vi "Camera Messenger.vi"(0 "Notifier Name":string, 2 "General Camera Actions":T3, 5 "Exposure Time (s)":dbl, 7 "Save Path":path, 9 "No. of Frames":u32, 11 "Camera ROI":T1, 12 "Cooler On/Off":bool, 13 "Defect Correction On/Off":bool, 14 "Fan On/Off":bool) -> (3 "Current Exposure Time (s)":dbl, 4 "Notifier Name Dup":string, 6 "Running?":bool, 8 "Camera ROI":T1, 10 "Current Frame":u32, 15 "Image Ref":T2)   [LabVIEW 2016]
uses:
  Camera Controls/Generic Camera Actions.ctl
  Camera Controls/Generic Camera ROI.ctl
  <vilib>/vision/Image Controls.llb/IMAQ Image.ctl
  Hardware Configuration/Hardware Configuration Controls/Company.ctl
  Hamamatsu/Orca Flash/Orca Flash Controls/Orca Flash ROI.ctl
  Hamamatsu/Orca Flash/Orca Flash Controls/Orca Flash Parameters.ctl
  Hamamatsu/Orca Flash/Orca Flash Controls/Orca Flash Parameter List.ctl
  Hamamatsu/Orca Flash/Orca Flash Controls/Orca Flash Actions.ctl
  IDS/IDS Controls/IDS ROI.ctl
  IDS/IDS Controls/IDS Parameters.ctl
  IDS/IDS Controls/IDS Parameter List.ctl
  IDS/IDS Controls/IDS Actions.ctl
  Photometrics/Prime BSI/Prime BSI Controls/Prime ROI.ctl
  Photometrics/Prime BSI/Prime BSI Controls/Prime Parameters.ctl
  Photometrics/Prime BSI/Prime BSI Controls/Prime Parameter List.ctl
  Photometrics/Prime BSI/Prime BSI Controls/Prime Actions.ctl
  Camera Controls/Camera IMAQ Key Info.ctl
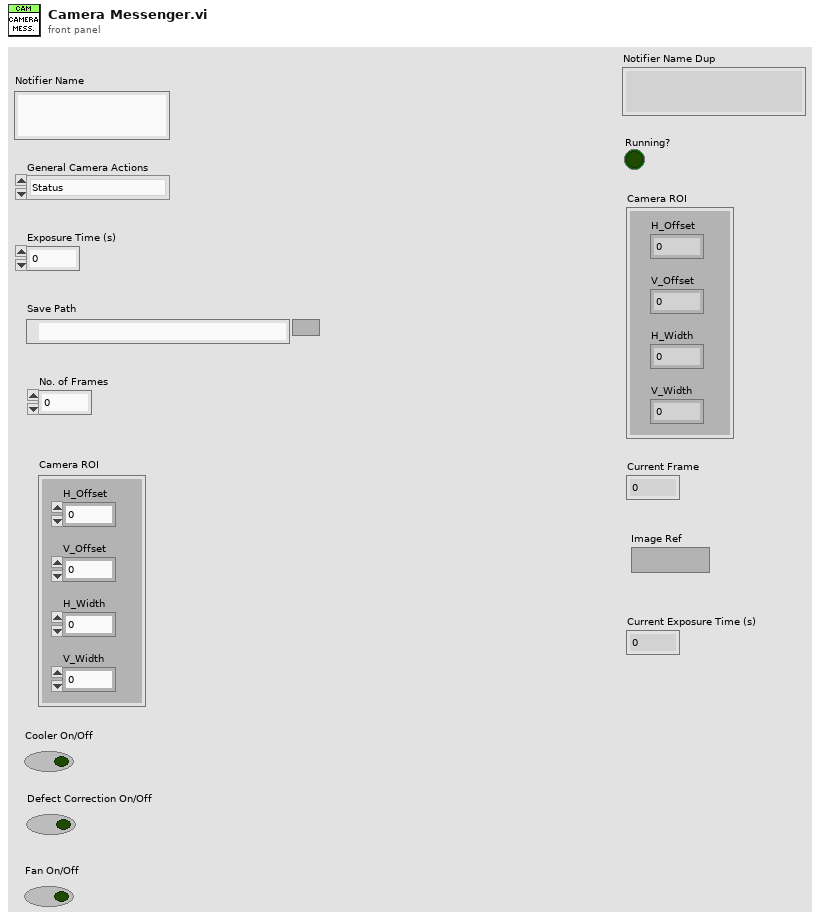
[diagram p1: front panel]
types:
  T1 = typedef "Generic Camera ROI.ctl" = cluster{"H_Offset":u16, "V_Offset":u16, "H_Width":u16, "V_Width":u16}
  T2 = typedef "IMAQ Image.ctl" = refnum<image>
  T3 = typedef "Generic Camera Actions.ctl" = enum16{"Status", "Ext trigger\n", "Live Preview", "Capture", "Abort", "Set Exposure Time (s)", "Get Exposure Time (s)", "Record Settings", "Set ROI", "Get ROI", "Defect Correction On/Off", "Cooler On/Off", "Fan On/Off", "Quti"}
  T4 = typedef "Company.ctl" = enum16{"AA Opto Electronic", "ASI", "Coherent", "CVI", "DAQmx", "Hamamatsu", "IDS", "Mad City Labs", "Marzhauser", "Measurement Computing", "MPB Com", "Photometrics", "PI", "Prior", "Thorlabs"}
  T5 = typedef "Orca Flash Parameters.ctl" = cluster{"Value":dbl, "Parameter":T6}
  T6 = typedef "Orca Flash Parameter List.ctl" = u32
  T7 = typedef "Orca Flash ROI.ctl" = cluster{"H Offset":i32, "V Offset":i32, "H Width":i32, "V Width":i32}
  T8 = typedef "Orca Flash Actions.ctl" = enum16{"IDLE", "PREVIEW", "RECORD", "Record Settings", "SETPARAM", "GETPARAM", "SETROI", "GETROI", "PROGRESSIVE MODE", "AREA MODE", "STATUS", "Trigger synchronous", "Trigger internal", "QUIT"}
  T9 = typedef "IDS Parameter List.ctl" = enum16{"Exposure Time (s)"}
  T10 = typedef "IDS Parameters.ctl" = cluster{"Parameter":T9, "Value":dbl}
  T11 = typedef "IDS ROI.ctl" = cluster{"H Offset":i32, "V Offset":i32, "H Width":i32, "V Width":i32}
  T12 = typedef "IDS Actions.ctl" = enum16{"Error Check", "Initialize", "Preview", "Record", "Abort", "Record Settings", "Set Parameter", "Get Parameter", "Set ROI", "Get ROI", "Status", "Quit"}
  T13 = typedef "Prime Parameter List.ctl" = enum16{"Exposure Time (s)"}
  T14 = typedef "Prime Parameters.ctl" = cluster{"Parameter":T13, "Value":dbl}
  T15 = typedef "Prime ROI.ctl" = cluster{"X Start":u32, "X End":u32, "X Bin":u32, "Y Start":u32, "Y End":u32, "Y Bin":u32}
  T16 = typedef "Prime Actions.ctl" = enum16{"Error Check", "Initialize", "Preview", "Record", "Abort", "Record Settings", "Set Parameter", "Get Parameter", "Set ROI", "Get ROI", "Status", "Set Trigger", "Quit"}
  T17 = typedef "Camera IMAQ Key Info.ctl" = cluster{"Frame":u32, "Sensor Height":i32, "Sensor Width":i32, "ROI Height":i32, "ROI Width":i32, "ROI Enable?":bool, "Bit per Pixel":u8}
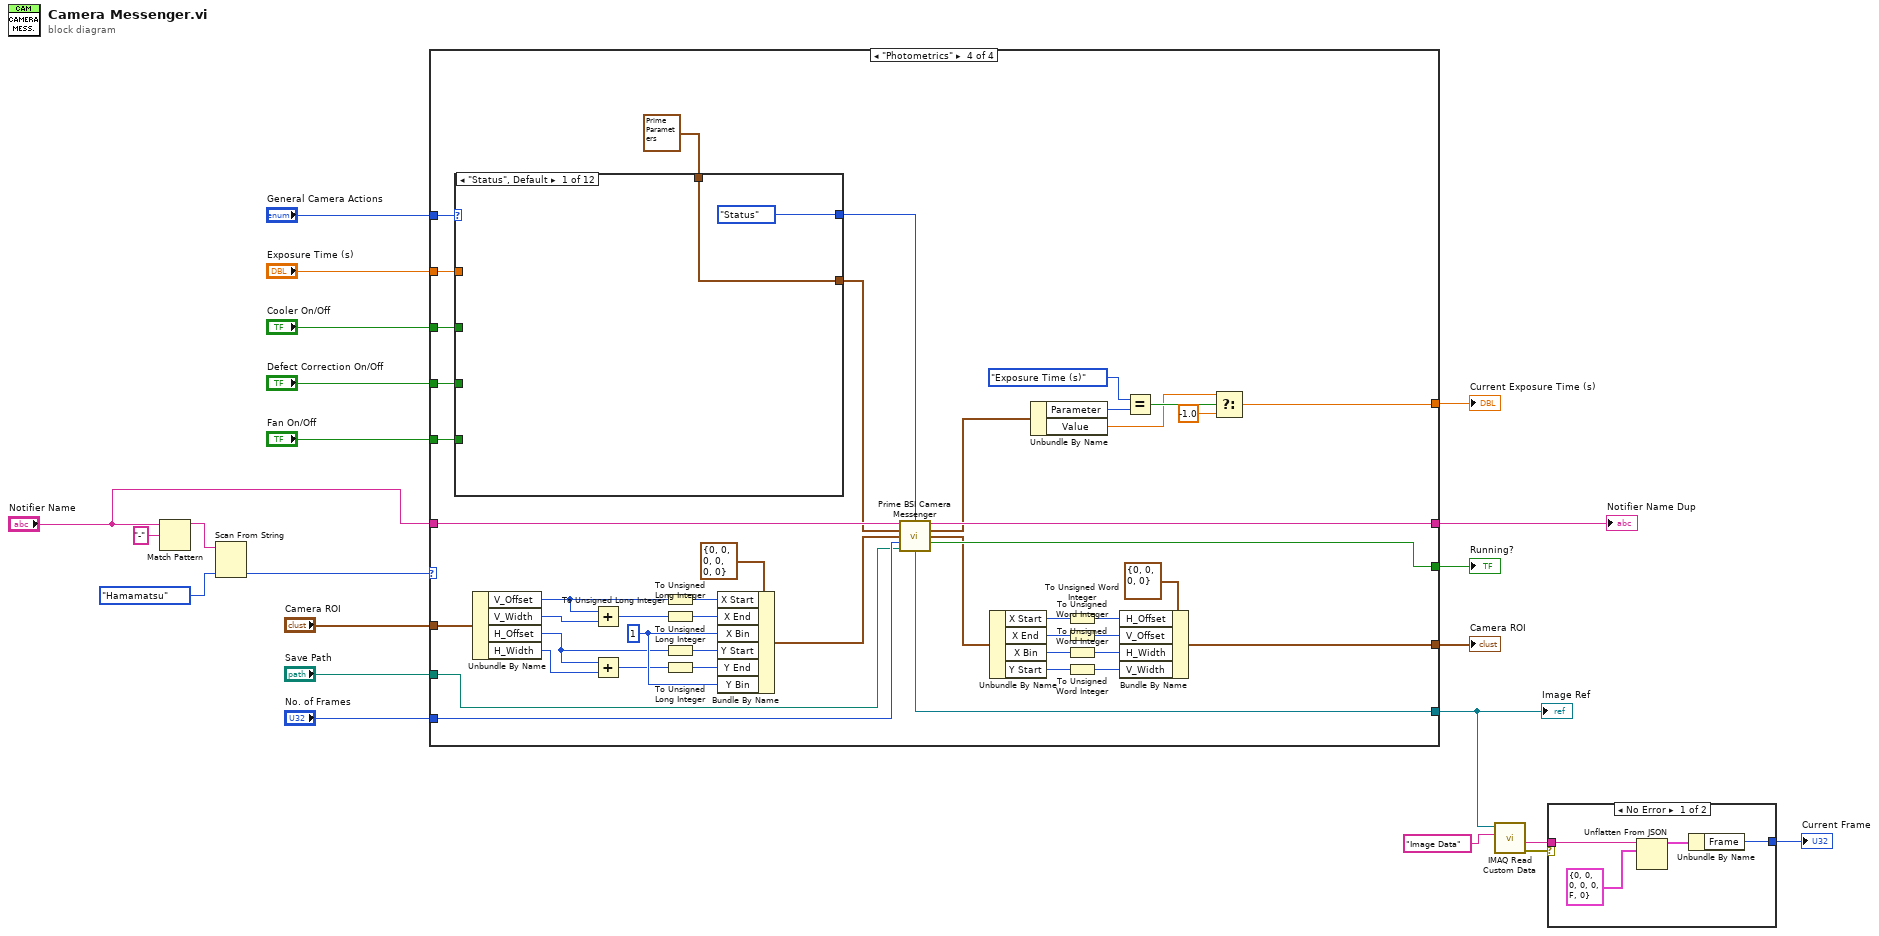
[diagram p0: block diagram]
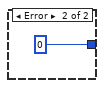
[diagram p2: hidden frame]
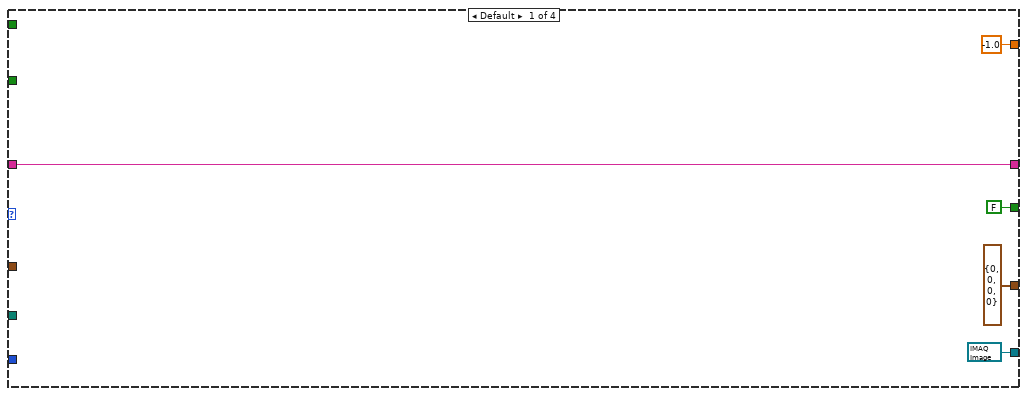
[diagram p3: hidden frame]
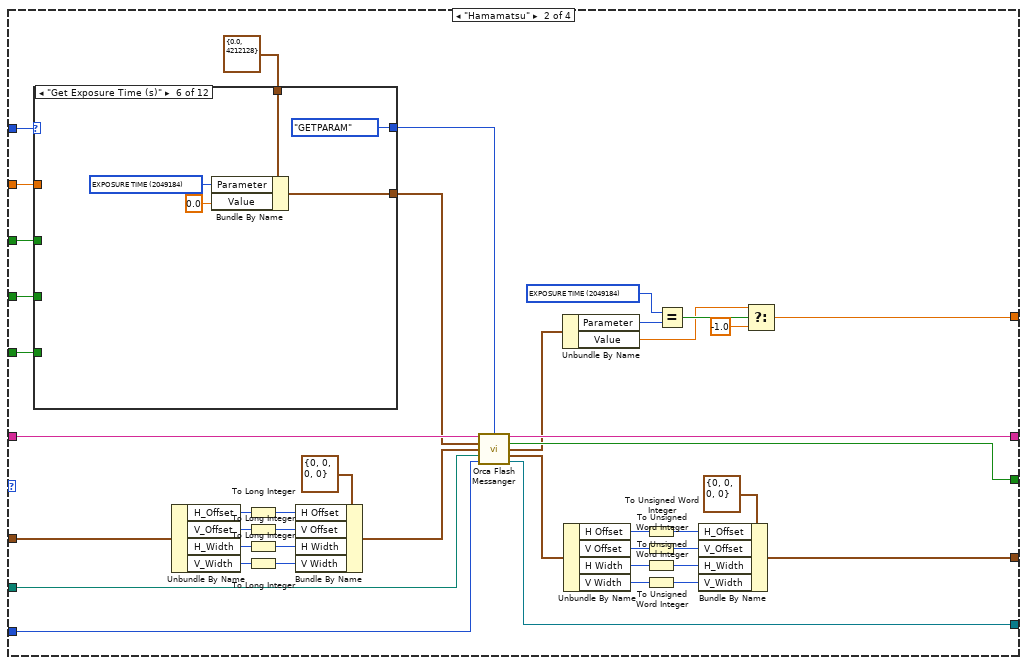
[diagram p4: hidden frame]
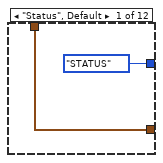
[diagram p5: hidden frame]
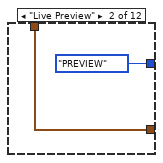
[diagram p6: hidden frame]
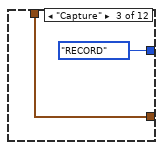
[diagram p7: hidden frame]
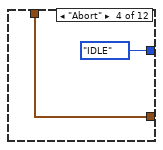
[diagram p8: hidden frame]
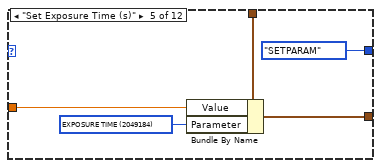
[diagram p9: hidden frame]
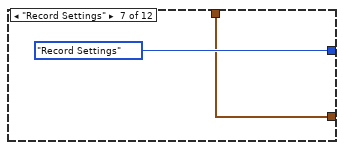
[diagram p10: hidden frame]
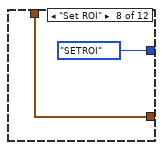
[diagram p11: hidden frame]
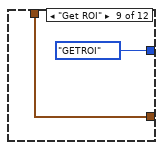
[diagram p12: hidden frame]
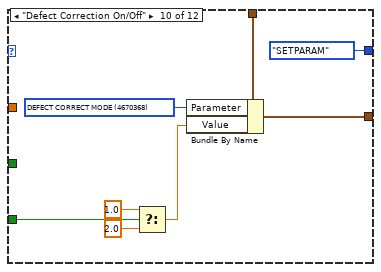
[diagram p13: hidden frame]
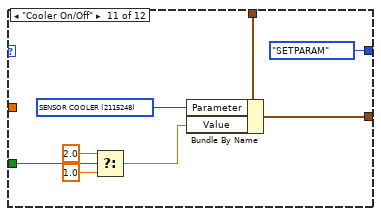
[diagram p14: hidden frame]
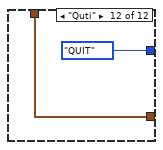
[diagram p15: hidden frame]
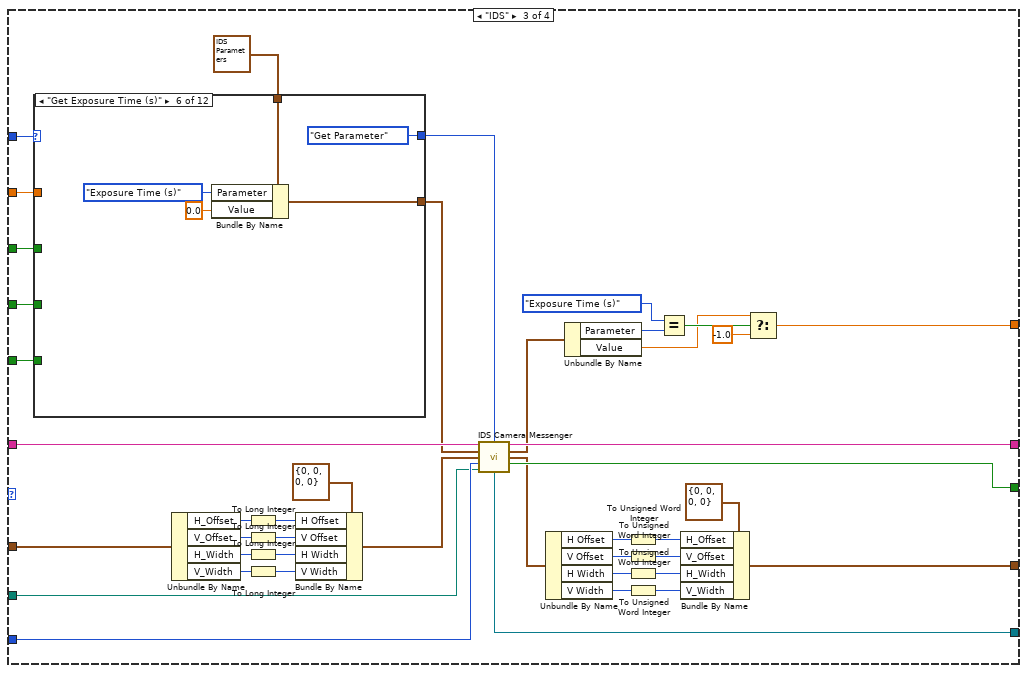
[diagram p16: hidden frame]
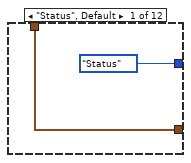
[diagram p17: hidden frame]
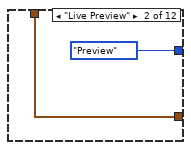
[diagram p18: hidden frame]
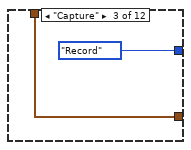
[diagram p19: hidden frame]
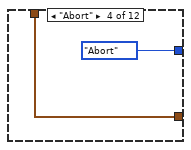
[diagram p20: hidden frame]
diagram:
  n1 = Match Pattern(string="Notifier Name", regular expression="-") -> (before substring=w19:string)  [unwired: 1 in, 3 out]
  n2 = Scan From String(input string=w19, default 1=Company."Hamamatsu" ("Company")) -> (output 1=w20:T4)  [unwired: 3 in, 3 out]
  n3 = case shown="\"Photometrics\"" w20 {
    tunnel: "Notifier Name" -> [w27 w70 w155 w231]
    tunnel: "General Camera Actions" -> [_ w55 w140 w224]
    tunnel: "No. of Frames" -> [_ w69 w154 w230]
    tunnel: "Save Path" -> [_ w68 w153 w202]
    tunnel: "Camera ROI" -> [_ w66 w151 w228]
    tunnel: [w27 w56 w141 w225] -> w14
    tunnel: "Exposure Time (s)" -> [_ w50 w136 w220]
    tunnel: "Cooler On/Off" -> [_ w54 w139 w223]
    tunnel: "Defect Correction On/Off" -> [_ w53 w138 w222]
    tunnel: "Fan On/Off" -> [_ w52 w137 w221]
    tunnel: [T2 refnum ("Image Ref") w47 w133 w217] -> w5
    tunnel: [FALSE ("Running?") w46 w132 w216] -> w9
    tunnel: [T1 {"H_Offset"=0, "V_Offset"=0, "H_Width"=0, "V_Width"=0} ("General Camera ROI") w35 w121 w205] -> w8
    tunnel: [-1.0 ("f") w29 w113 w187] -> w1
    frame Default {
    }
    frame "Hamamatsu" {
      w28 = T6 2049184 items=["SENSOR MODE"=4212128, "READOUT SPEED"=4211872, "READOUT DIRECTION"=4211904, "TRIGGER GLOBAL EXPOSURE"=2049680, "TRIGGER DELAY"=1066480, "SYNC READOUT SYSTEM BLANK"=1066528, "SENSOR COOLER"=2115248, "SENSOR COOLER STATUS"=2115280, "EXPOSURE TIME"=2049184, "DEFECT CORRECT MODE"=4670368, "BINNING"=4215968, "INTERNAL LINE SPEED"=4226000, "INTERNAL LINE INTERVAL"=4226016, "IMAGE PIXEL TYPE"=4343296, "NUMBER OF OUTPUT TRIGGER CONNECTOR"=1852320, "OUTPUT TRIGGER SOURCE[0]"=1852576, "OUTPUT TRIGGER SOURCE[1]"=1852832, "OUTPUT TRIGGER SOURCE[2]"=1853088, "OUTPUT TRIGGER POLARITY[0]"=1852592, "OUTPUT TRIGGER POLARITY[1]"=1852848, "OUTPUT TRIGGER POLARITY[2]"=1853104, "OUTPUT TRIGGER ACTIVE[0]"=1852608, "OUTPUT TRIGGER ACTIVE[1]"=1852864, "OUTPUT TRIGGER ACTIVE[2]"=1853120, "OUTPUT TRIGGER DELAY[0]"=1852624, "OUTPUT TRIGGER DELAY[1]"=1852880, "OUTPUT TRIGGER DELAY[2]"=1853136, "OUTPUT TRIGGER PERIOD[0]"=1852640, "OUTPUT TRIGGER PERIOD[1]"=1852896, "OUTPUT TRIGGER PERIOD[2]"=1853152, "OUTPUT TRIGGER KIND[0]"=1852656, "OUTPUT TRIGGER KIND[1]"=1852912, "OUTPUT TRIGGER KIND[2]"=1853168, "OUTPUT TRIGGER PRE HSYNC COUNT"=1852704] ("x")
      n4 = case shown="\"Get Exposure Time (s)\"" w55 {
        tunnel: w54 -> [_ _ _ _ _ _ _ _ _ _ w107 _]
        tunnel: w53 -> [_ _ _ _ _ _ _ _ _ w98 _ _]
        tunnel: w52 -> [_ _ _ _ _ _ _ _ _ _ _ _]
        tunnel: [Orca_Flash_Actions."STATUS" ("Camera Actions") Orca_Flash_Actions."PREVIEW" ("Camera Actions") Orca_Flash_Actions."RECORD" ("Camera Actions") Orca_Flash_Actions."IDLE" ("Camera Actions") Orca_Flash_Actions."SETPARAM" ("Camera Actions") Orca_Flash_Actions."GETPARAM" ("Camera Actions") Orca_Flash_Actions."Record Settings" ("Camera Actions") Orca_Flash_Actions."SETROI" ("Camera Actions") Orca_Flash_Actions."GETROI" ("Camera Actions") Orca_Flash_Actions."SETPARAM" ("Camera Actions") Orca_Flash_Actions."SETPARAM" ("Camera Actions") Orca_Flash_Actions."QUIT" ("Camera Actions")] -> w51
        tunnel: w50 -> [_ _ _ _ w82 _ _ _ _ _ _ _]
        tunnel: [w71 w73 w75 w77 w81 w87 w89 w91 w93 w100 w103 w112] -> w49
        tunnel: T5 {"Value"=0.0, "Parameter"=4212128} ("sCMOS Parameter") -> [w71 w73 w75 w77 w80 w88 w89 w91 w93 w101 w109 w112]
        frame "Status", Default {
        }
        frame "Live Preview" {
        }
        frame "Capture" {
        }
        frame "Abort" {
        }
        frame "Set Exposure Time (s)" {
          w79 = T6 2049184 items=["SENSOR MODE"=4212128, "READOUT SPEED"=4211872, "READOUT DIRECTION"=4211904, "TRIGGER GLOBAL EXPOSURE"=2049680, "TRIGGER DELAY"=1066480, "SYNC READOUT SYSTEM BLANK"=1066528, "SENSOR COOLER"=2115248, "SENSOR COOLER STATUS"=2115280, "EXPOSURE TIME"=2049184, "DEFECT CORRECT MODE"=4670368, "BINNING"=4215968, "INTERNAL LINE SPEED"=4226000, "INTERNAL LINE INTERVAL"=4226016, "IMAGE PIXEL TYPE"=4343296, "NUMBER OF OUTPUT TRIGGER CONNECTOR"=1852320, "OUTPUT TRIGGER SOURCE[0]"=1852576, "OUTPUT TRIGGER SOURCE[1]"=1852832, "OUTPUT TRIGGER SOURCE[2]"=1853088, "OUTPUT TRIGGER POLARITY[0]"=1852592, "OUTPUT TRIGGER POLARITY[1]"=1852848, "OUTPUT TRIGGER POLARITY[2]"=1853104, "OUTPUT TRIGGER ACTIVE[0]"=1852608, "OUTPUT TRIGGER ACTIVE[1]"=1852864, "OUTPUT TRIGGER ACTIVE[2]"=1853120, "OUTPUT TRIGGER DELAY[0]"=1852624, "OUTPUT TRIGGER DELAY[1]"=1852880, "OUTPUT TRIGGER DELAY[2]"=1853136, "OUTPUT TRIGGER PERIOD[0]"=1852640, "OUTPUT TRIGGER PERIOD[1]"=1852896, "OUTPUT TRIGGER PERIOD[2]"=1853152, "OUTPUT TRIGGER KIND[0]"=1852656, "OUTPUT TRIGGER KIND[1]"=1852912, "OUTPUT TRIGGER KIND[2]"=1853168, "OUTPUT TRIGGER PRE HSYNC COUNT"=1852704] ("Parameter")
          n5 = Bundle By Name(cluster=w80, "Value"=w82, "Parameter"=w79) -> (w81:T5)
        }
        frame "Get Exposure Time (s)" {
          w85 = T6 2049184 items=["SENSOR MODE"=4212128, "READOUT SPEED"=4211872, "READOUT DIRECTION"=4211904, "TRIGGER GLOBAL EXPOSURE"=2049680, "TRIGGER DELAY"=1066480, "SYNC READOUT SYSTEM BLANK"=1066528, "SENSOR COOLER"=2115248, "SENSOR COOLER STATUS"=2115280, "EXPOSURE TIME"=2049184, "DEFECT CORRECT MODE"=4670368, "BINNING"=4215968, "INTERNAL LINE SPEED"=4226000, "INTERNAL LINE INTERVAL"=4226016, "IMAGE PIXEL TYPE"=4343296, "NUMBER OF OUTPUT TRIGGER CONNECTOR"=1852320, "OUTPUT TRIGGER SOURCE[0]"=1852576, "OUTPUT TRIGGER SOURCE[1]"=1852832, "OUTPUT TRIGGER SOURCE[2]"=1853088, "OUTPUT TRIGGER POLARITY[0]"=1852592, "OUTPUT TRIGGER POLARITY[1]"=1852848, "OUTPUT TRIGGER POLARITY[2]"=1853104, "OUTPUT TRIGGER ACTIVE[0]"=1852608, "OUTPUT TRIGGER ACTIVE[1]"=1852864, "OUTPUT TRIGGER ACTIVE[2]"=1853120, "OUTPUT TRIGGER DELAY[0]"=1852624, "OUTPUT TRIGGER DELAY[1]"=1852880, "OUTPUT TRIGGER DELAY[2]"=1853136, "OUTPUT TRIGGER PERIOD[0]"=1852640, "OUTPUT TRIGGER PERIOD[1]"=1852896, "OUTPUT TRIGGER PERIOD[2]"=1853152, "OUTPUT TRIGGER KIND[0]"=1852656, "OUTPUT TRIGGER KIND[1]"=1852912, "OUTPUT TRIGGER KIND[2]"=1853168, "OUTPUT TRIGGER PRE HSYNC COUNT"=1852704] ("Parameter")
          n6 = Bundle By Name(cluster=w88, "Parameter"=w85, "Value"=0.0) -> (w87:T5)
        }
        frame "Record Settings" {
        }
        frame "Set ROI" {
        }
        frame "Get ROI" {
        }
        frame "Defect Correction On/Off" {
          w99 = T6 4670368 items=["SENSOR MODE"=4212128, "READOUT SPEED"=4211872, "READOUT DIRECTION"=4211904, "TRIGGER GLOBAL EXPOSURE"=2049680, "TRIGGER DELAY"=1066480, "SYNC READOUT SYSTEM BLANK"=1066528, "SENSOR COOLER"=2115248, "SENSOR COOLER STATUS"=2115280, "EXPOSURE TIME"=2049184, "DEFECT CORRECT MODE"=4670368, "BINNING"=4215968, "INTERNAL LINE SPEED"=4226000, "INTERNAL LINE INTERVAL"=4226016, "IMAGE PIXEL TYPE"=4343296, "NUMBER OF OUTPUT TRIGGER CONNECTOR"=1852320, "OUTPUT TRIGGER SOURCE[0]"=1852576, "OUTPUT TRIGGER SOURCE[1]"=1852832, "OUTPUT TRIGGER SOURCE[2]"=1853088, "OUTPUT TRIGGER POLARITY[0]"=1852592, "OUTPUT TRIGGER POLARITY[1]"=1852848, "OUTPUT TRIGGER POLARITY[2]"=1853104, "OUTPUT TRIGGER ACTIVE[0]"=1852608, "OUTPUT TRIGGER ACTIVE[1]"=1852864, "OUTPUT TRIGGER ACTIVE[2]"=1853120, "OUTPUT TRIGGER DELAY[0]"=1852624, "OUTPUT TRIGGER DELAY[1]"=1852880, "OUTPUT TRIGGER DELAY[2]"=1853136, "OUTPUT TRIGGER PERIOD[0]"=1852640, "OUTPUT TRIGGER PERIOD[1]"=1852896, "OUTPUT TRIGGER PERIOD[2]"=1853152, "OUTPUT TRIGGER KIND[0]"=1852656, "OUTPUT TRIGGER KIND[1]"=1852912, "OUTPUT TRIGGER KIND[2]"=1853168, "OUTPUT TRIGGER PRE HSYNC COUNT"=1852704] ("Parameter")
          n7 = Select(t=1.0, s=w98, f=2.0) -> (s? t:f=w95:dbl)
          n8 = Bundle By Name(cluster=w101, "Parameter"=w99, "Value"=w95) -> (w100:T5)
        }
        frame "Cooler On/Off" {
          w108 = T6 2115248 items=["SENSOR MODE"=4212128, "READOUT SPEED"=4211872, "READOUT DIRECTION"=4211904, "TRIGGER GLOBAL EXPOSURE"=2049680, "TRIGGER DELAY"=1066480, "SYNC READOUT SYSTEM BLANK"=1066528, "SENSOR COOLER"=2115248, "SENSOR COOLER STATUS"=2115280, "EXPOSURE TIME"=2049184, "DEFECT CORRECT MODE"=4670368, "BINNING"=4215968, "INTERNAL LINE SPEED"=4226000, "INTERNAL LINE INTERVAL"=4226016, "IMAGE PIXEL TYPE"=4343296, "NUMBER OF OUTPUT TRIGGER CONNECTOR"=1852320, "OUTPUT TRIGGER SOURCE[0]"=1852576, "OUTPUT TRIGGER SOURCE[1]"=1852832, "OUTPUT TRIGGER SOURCE[2]"=1853088, "OUTPUT TRIGGER POLARITY[0]"=1852592, "OUTPUT TRIGGER POLARITY[1]"=1852848, "OUTPUT TRIGGER POLARITY[2]"=1853104, "OUTPUT TRIGGER ACTIVE[0]"=1852608, "OUTPUT TRIGGER ACTIVE[1]"=1852864, "OUTPUT TRIGGER ACTIVE[2]"=1853120, "OUTPUT TRIGGER DELAY[0]"=1852624, "OUTPUT TRIGGER DELAY[1]"=1852880, "OUTPUT TRIGGER DELAY[2]"=1853136, "OUTPUT TRIGGER PERIOD[0]"=1852640, "OUTPUT TRIGGER PERIOD[1]"=1852896, "OUTPUT TRIGGER PERIOD[2]"=1853152, "OUTPUT TRIGGER KIND[0]"=1852656, "OUTPUT TRIGGER KIND[1]"=1852912, "OUTPUT TRIGGER KIND[2]"=1853168, "OUTPUT TRIGGER PRE HSYNC COUNT"=1852704] ("Parameter")
          n9 = Select(t=2.0, s=w107, f=1.0) -> (s? t:f=w104:dbl)
          n10 = Bundle By Name(cluster=w109, "Parameter"=w108, "Value"=w104) -> (w103:T5)
        }
        frame "Quti" {
        }
      }
      n11 = Unbundle By Name(w66) -> ("H_Offset"=w62:u16, "V_Offset"=w63:u16, "H_Width"=w64:u16, "V_Width"=w65:u16)
      n12 = To Long Integer(number=w62) -> (32bit integer=w61:i32)
      n13 = To Long Integer(number=w63) -> (32bit integer=w60:i32)
      n14 = To Long Integer(number=w64) -> (32bit integer=w59:i32)
      n15 = To Long Integer(number=w65) -> (32bit integer=w58:i32)
      n16 = Bundle By Name(cluster=T7 {"H Offset"=0, "V Offset"=0, "H Width"=0, "V Width"=0} ("sCMOS ROI"), "H Offset"=w61, "V Offset"=w60, "H Width"=w59, "V Width"=w58) -> (w57:T7)
      n17 = call "Orca Flash Messanger.vi"("Notifier Name"=w70, "Camera Actions"=w51, "sCMOS Parameter"=w49, "sCMOS ROI"=w57, "Path"=w68, "# of frames"=w69) -> ("Notifier Name Dup"=w56:string, "Running?"=w46:bool, "sCMOS Parameter"=w30:T5, "sCMOS ROI"=w44:T7, "Image Ref"=w47:T2)  [unwired: 5 in]
      n18 = Unbundle By Name(w30) -> ("Parameter"=w34:T6, "Value"=w32:dbl)
      n19 = Unbundle By Name(w44) -> ("H Offset"=w43:i32, "V Offset"=w42:i32, "H Width"=w41:i32, "V Width"=w40:i32)
      n20 = To Unsigned Word Integer(number=w43) -> (unsigned 16bit integer=w39:u16)
      n21 = To Unsigned Word Integer(number=w42) -> (unsigned 16bit integer=w38:u16)
      n22 = To Unsigned Word Integer(number=w41) -> (unsigned 16bit integer=w37:u16)
      n23 = To Unsigned Word Integer(number=w40) -> (unsigned 16bit integer=w36:u16)
      n24 = Equal?(x=w28, y=w34) -> (x = y?=w33:bool)
      n25 = Bundle By Name(cluster=T1 {"H_Offset"=0, "V_Offset"=0, "H_Width"=0, "V_Width"=0} ("General Camera ROI"), "H_Offset"=w39, "V_Offset"=w38, "H_Width"=w37, "V_Width"=w36) -> (w35:T1)
      n26 = Select(t=w32, s=w33, f=-1.0) -> (s? t:f=w29:dbl)
    }
    frame "IDS" {
      n27 = case shown="\"Get Exposure Time (s)\"" w140 {
        tunnel: w139 -> [_ _ _ _ _ _ _ _ _ _ _ _]
        tunnel: w138 -> [_ _ _ _ _ _ _ _ _ _ _ _]
        tunnel: w137 -> [_ _ _ _ _ _ _ _ _ _ _ _]
        tunnel: [IDS_Actions."Status" ("IDS Actions") IDS_Actions."Preview" ("IDS Actions") IDS_Actions."Record" ("IDS Actions") IDS_Actions."Abort" ("IDS Actions") IDS_Actions."Set Parameter" ("IDS Actions") IDS_Actions."Get Parameter" ("IDS Actions") IDS_Actions."Record Settings" ("IDS Actions") IDS_Actions."Set ROI" ("IDS Actions") IDS_Actions."Get ROI" ("IDS Actions") IDS_Actions."Status" ("IDS Actions") IDS_Actions."Status" ("IDS Actions") IDS_Actions."Quit" ("IDS Actions")] -> w120
        tunnel: w136 -> [_ _ _ _ w168 _ _ _ _ _ _ _]
        tunnel: [w157 w159 w161 w163 w167 w169 w175 w177 w179 w181 w183 w185] -> w135
        tunnel: T10 {"Parameter"=enum."Exposure Time (s)", "Value"=4212128.0} ("IDS Parameter") -> [w157 w159 w161 w163 w166 w172 w175 w177 w179 w181 w183 w185]
        frame "Status", Default {
        }
        frame "Live Preview" {
        }
        frame "Capture" {
        }
        frame "Abort" {
        }
        frame "Set Exposure Time (s)" {
          n28 = Bundle By Name(cluster=w166, "Value"=w168, "Parameter"=IDS_Parameter_List."Exposure Time (s)") -> (w167:T10)
        }
        frame "Get Exposure Time (s)" {
          n29 = Bundle By Name(cluster=w172, "Parameter"=IDS_Parameter_List."Exposure Time (s)", "Value"=0.0) -> (w169:T10)
        }
        frame "Record Settings" {
        }
        frame "Set ROI" {
        }
        frame "Get ROI" {
        }
        frame "Defect Correction On/Off" {
        }
        frame "Cooler On/Off" {
        }
        frame "Quti" {
        }
      }
      n30 = Unbundle By Name(w151) -> ("H_Offset"=w147:u16, "V_Offset"=w148:u16, "H_Width"=w149:u16, "V_Width"=w150:u16)
      n31 = To Long Integer(number=w147) -> (32bit integer=w146:i32)
      n32 = To Long Integer(number=w148) -> (32bit integer=w145:i32)
      n33 = To Long Integer(number=w149) -> (32bit integer=w144:i32)
      n34 = To Long Integer(number=w150) -> (32bit integer=w143:i32)
      n35 = Bundle By Name(cluster=T11 {"H Offset"=0, "V Offset"=0, "H Width"=0, "V Width"=0} ("sCMOS ROI"), "H Offset"=w146, "V Offset"=w145, "H Width"=w144, "V Width"=w143) -> (w142:T11)
      n36 = call "IDS Camera Messenger.vi"("Notifier Name"=w155, "IDS Actions"=w120, "IDS Parameter"=w135, "ROI Setup"=w142, "# of Frames"=w154, "File Save Path"=w153) -> ("Notifier Name (Dup)"=w141:string, "IDS Parameter"=w119:T10, "IDS ROI"=w130:T11, "Running?"=w132:bool, "Image Ref"=w133:T2)  [unwired: 4 in, 1 out]
      n37 = Unbundle By Name(w130) -> ("H Offset"=w129:i32, "V Offset"=w128:i32, "H Width"=w127:i32, "V Width"=w126:i32)
      n38 = Unbundle By Name(w119) -> ("Parameter"=w118:T9, "Value"=w115:dbl)
      n39 = To Unsigned Word Integer(number=w129) -> (unsigned 16bit integer=w125:u16)
      n40 = To Unsigned Word Integer(number=w128) -> (unsigned 16bit integer=w124:u16)
      n41 = To Unsigned Word Integer(number=w127) -> (unsigned 16bit integer=w123:u16)
      n42 = To Unsigned Word Integer(number=w126) -> (unsigned 16bit integer=w122:u16)
      n43 = Equal?(x=IDS_Parameter_List."Exposure Time (s)", y=w118) -> (x = y?=w116:bool)
      n44 = Bundle By Name(cluster=T1 {"H_Offset"=0, "V_Offset"=0, "H_Width"=0, "V_Width"=0} ("General Camera ROI"), "H_Offset"=w125, "V_Offset"=w124, "H_Width"=w123, "V_Width"=w122) -> (w121:T1)
      n45 = Select(t=w115, s=w116, f=-1.0) -> (s? t:f=w113:dbl)
    }
    frame "Photometrics" {
      w203 = u32 1 ("number")
      n46 = case shown="\"Status\", Default" w224 {
        tunnel: w223 -> [_ _ _ _ _ _ _ _ _ _ _ _]
        tunnel: w222 -> [_ _ _ _ _ _ _ _ _ _ _ _]
        tunnel: w221 -> [_ _ _ _ _ _ _ _ _ _ _ _]
        tunnel: [Prime_Actions."Status" ("Prime Actions") Prime_Actions."Preview" ("Prime Actions") Prime_Actions."Record" ("Prime Actions") Prime_Actions."Abort" ("Prime Actions") Prime_Actions."Set Parameter" ("Prime Actions") Prime_Actions."Get Parameter" ("Prime Actions") Prime_Actions."Record Settings" ("Prime Actions") Prime_Actions."Set ROI" ("Prime Actions") Prime_Actions."Get ROI" ("Prime Actions") Prime_Actions."Status" ("Prime Actions") Prime_Actions."Status" ("Prime Actions") Prime_Actions."Quit" ("Prime Actions")] -> w204
        tunnel: w220 -> [_ _ _ _ w244 _ _ _ _ _ _ _]
        tunnel: [w233 w235 w237 w239 w243 w247 w251 w253 w255 w257 w259 w261] -> w219
        tunnel: T14 {"Parameter"=enum."Exposure Time (s)", "Value"=4212128.0} ("Prime Parameter") -> [w233 w235 w237 w239 w242 w248 w251 w253 w255 w257 w259 w261]
        frame "Status", Default {
        }
        frame "Live Preview" {
        }
        frame "Capture" {
        }
        frame "Abort" {
        }
        frame "Set Exposure Time (s)" {
          n47 = Bundle By Name(cluster=w242, "Value"=w244, "Parameter"=Prime_Parameter_List."Exposure Time (s)") -> (w243:T14)
        }
        frame "Get Exposure Time (s)" {
          n48 = Bundle By Name(cluster=w248, "Parameter"=Prime_Parameter_List."Exposure Time (s)", "Value"=0.0) -> (w247:T14)
        }
        frame "Record Settings" {
        }
        frame "Set ROI" {
        }
        frame "Get ROI" {
        }
        frame "Defect Correction On/Off" {
        }
        frame "Cooler On/Off" {
        }
        frame "Quti" {
        }
      }
      n49 = Unbundle By Name(w228) -> ("V_Offset"=w194:u16, "V_Width"=w196:u16, "H_Offset"=w200:u16, "H_Width"=w201:u16)
      n50 = Add(x=w194, y=w196) -> (x+y=w195:u16)
      n51 = Add(x=w200, y=w201) -> (x+y=w198:u16)
      n52 = To Unsigned Long Integer(number=w194) -> (unsigned 32bit integer=w193:u32)
      n53 = To Unsigned Long Integer(number=w195) -> (unsigned 32bit integer=w227:u32)
      n54 = To Unsigned Long Integer(number=w200) -> (unsigned 32bit integer=w199:u32)
      n55 = To Unsigned Long Integer(number=w198) -> (unsigned 32bit integer=w197:u32)
      n56 = Bundle By Name(cluster=T15 {"X Start"=0, "X End"=0, "X Bin"=0, "Y Start"=0, "Y End"=0, "Y Bin"=0} ("sCMOS ROI"), "X Start"=w193, "X End"=w227, "X Bin"=w203, "Y Start"=w199, "Y End"=w197, "Y Bin"=w203) -> (w226:T15)
      n57 = call "Prime BSI Camera Messenger.vi"("Notifier Name"=w231, "Prime Actions"=w204, "Prime Parameter"=w219, "ROI Setup"=w226, "# of Frames"=w230, "File Save Path"=w202) -> ("Notifier Name (Dup)"=w225:string, "Prime Parameter"=w188:T14, "Prime ROI"=w214:T15, "Running?"=w216:bool, "Image Ref"=w217:T2)  [unwired: 4 in, 1 out]
      n58 = Unbundle By Name(w214) -> ("X Start"=w213:u32, "X End"=w212:u32, "X Bin"=w211:u32, "Y Start"=w210:u32)
      n59 = Unbundle By Name(w188) -> ("Parameter"=w192:T13, "Value"=w190:dbl)
      n60 = To Unsigned Word Integer(number=w213) -> (unsigned 16bit integer=w209:u16)
      n61 = To Unsigned Word Integer(number=w212) -> (unsigned 16bit integer=w208:u16)
      n62 = To Unsigned Word Integer(number=w211) -> (unsigned 16bit integer=w207:u16)
      n63 = To Unsigned Word Integer(number=w210) -> (unsigned 16bit integer=w206:u16)
      n64 = Bundle By Name(cluster=T1 {"H_Offset"=0, "V_Offset"=0, "H_Width"=0, "V_Width"=0} ("General Camera ROI"), "H_Offset"=w209, "V_Offset"=w208, "H_Width"=w207, "V_Width"=w206) -> (w205:T1)
      n65 = Equal?(x=Prime_Parameter_List."Exposure Time (s)", y=w192) -> (x = y?=w191:bool)
      n66 = Select(t=w190, s=w191, f=-1.0) -> (s? t:f=w187:dbl)
    }
  }
  "Notifier Name Dup" <- w14
  "Image Ref" <- w5
  "Running?" <- w9
  "Camera ROI" <- w8
  "Current Exposure Time (s)" <- w1
  n67 = call "IMAQ Read Custom Data"("Key"="Image Data", "Image"=w5) -> ("error out"=w4:errorcluster, "Custom Data Out"=w6:string)  [unwired: 7 in, 1 out]
  n68 = case shown="No Error" w4 {
    tunnel: w6 -> [w265 _]
    tunnel: [w262 u32 0 ("Frame")] -> w3
    frame No Error {
      n69 = Unflatten From JSON(JSON string=w265, type and defaults=T17 {"Frame"=0, "Sensor Height"=0, "Sensor Width"=0, "ROI Height"=0, "ROI Width"=0, "ROI Enable?"=FALSE, "Bit per Pixel"=0} ("Camera IMAQ Key Info")) -> (value=w263:T17)  [unwired: 5 in, 1 out]
      n70 = Unbundle By Name(w263) -> ("Frame"=w262:u32)
    }
    frame Error {
    }
  }
  "Current Frame" <- w3
